vi "P4CMD Dialog - Project Options.vi"(6 "operation message":string, 8 "error in (no error)":errorcluster, 9 "configuration data in":string) -> (0 "error out":errorcluster, 1 "configuration data out":string, 5 "cancelled?":bool)   [LabVIEW 2017, in "NI_SCC_P4CMD.lvlib"]
uses:
  <vilib>/SourceControl/Providers/P4CMD/NI_SCC_P4CMD.lvlib
  <vilib>/SourceControl/support/SCCSup Dialog_GenMCLB_OnlineHelp.ctl
  <vilib>/SourceControl/Providers/P4CMD/P4CMD Operations.ctl
  <vilib>/SourceControl/support/SCCSup Dialog_GenMCLB_FilterParams.ctl
  <vilib>/SourceControl/support/SCCSup Message Strings GLBL.vi
panel:
  in  "P4Proj UIDialog FP Refs":T1
  in  "use defaults":bool=TRUE
  in  "browse clients":bool
  in  "browse users":bool
  in  "Client Workspace":string
  in  "Password":string
  in  "User":string
  in  "Port":string
  in  "Server":string
  in  "OK":bool
  in  "Cancel":bool
  in  "Help":bool
  # "1"
  # "Connect to"
  # "2"
  # "Connect as"
  # "3"
  # "Open client workspace"
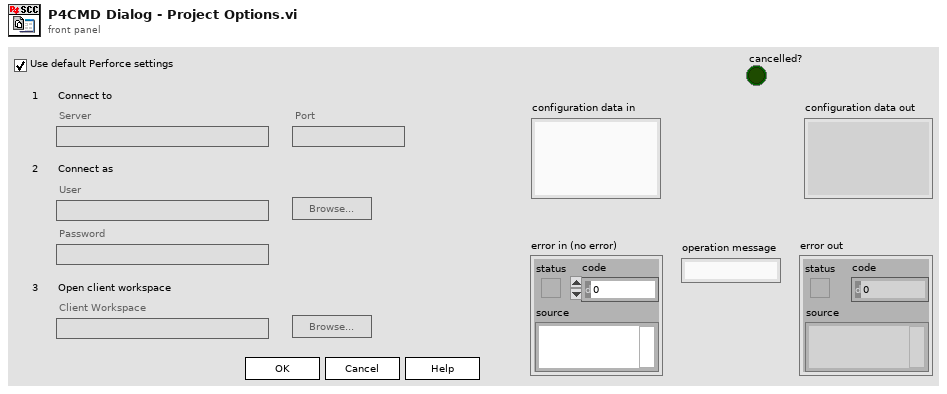
[diagram p1: front panel]
types:
  T1 = cluster{"browse users":refnum<vi>, "browse clients":refnum<vi>, "Server:":refnum<vi>, "Port:":refnum<vi>, "User:":refnum<vi>, "Password:":refnum<vi>, "Client Workspace:":refnum<vi>, "use default":refnum<vi>, "OK":refnum<vi>}
  T2 = typedef "SCCSup Dialog_GenMCLB_OnlineHelp.ctl" = cluster{"Operation":enum16{"Contents", "Key", "Close"}, "String to search for":string, "Path to the help file":path}
  T3 = typedef "NI_SCC_P4CMD.lvlib/P4CMD Operations.ctl" = enum16{"get all clients", "get all users", "describe changelist", "sync from depot", "open for edit", "submit to depot", "revert", "add to depot", "remove from depot", "print files revisions", "compare client file", "print depot file contents", "list opened files", "get file info", "lock files", "edit changelist spec", "info", "set variables"}
  T4 = typedef "SCCSup Dialog_GenMCLB_FilterParams.ctl" = cluster{"checkbox visible?":bool, "boolean text":string, "filter string":string, "filter column":i32}
  T5 = enum32{"Invalid", "Standard", "Closed", "Hidden", "Minimized", "Maximized"}
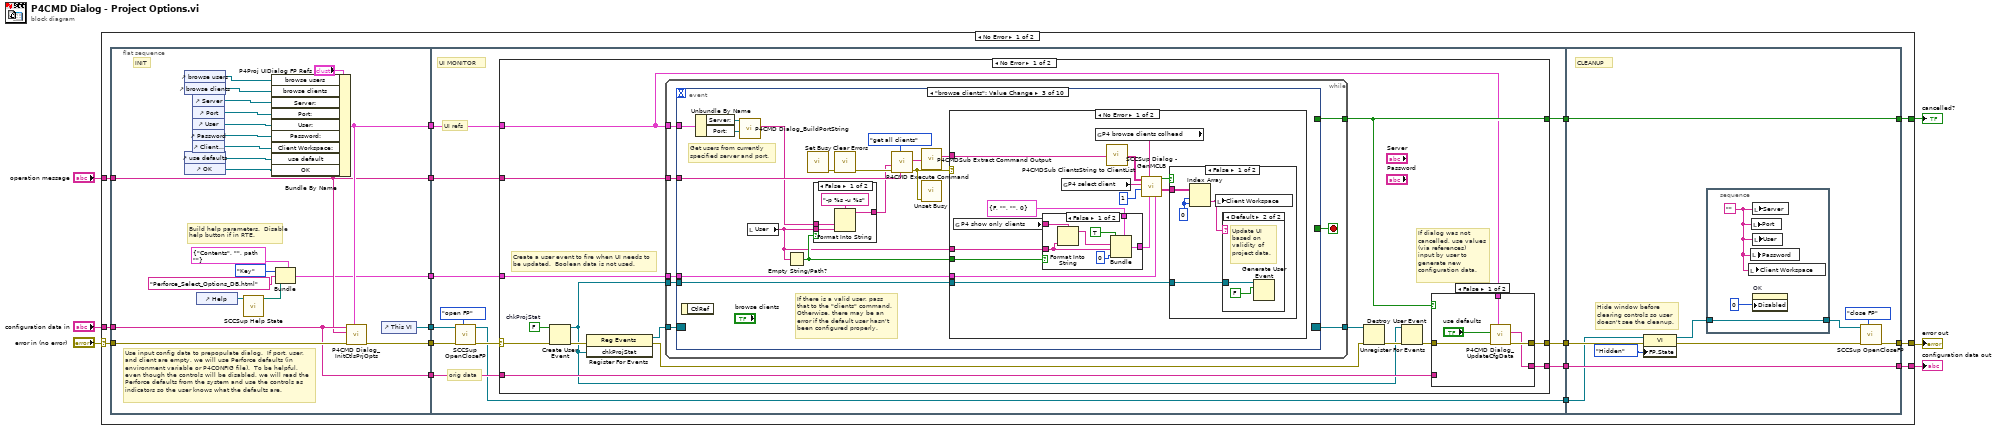
[diagram p0: block diagram]
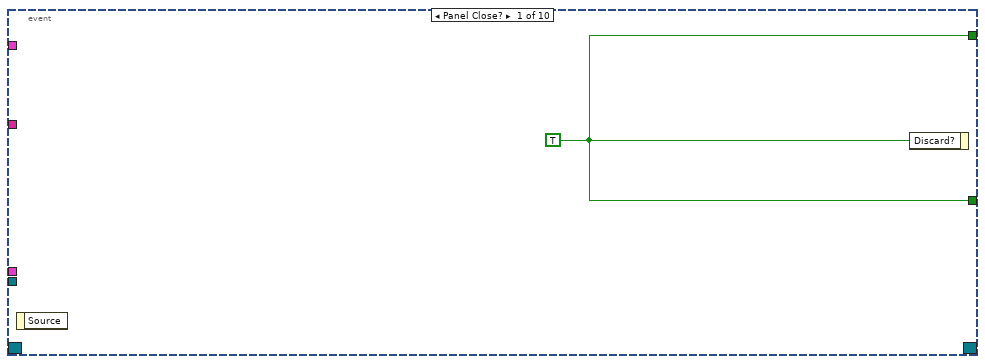
[diagram p3: hidden frame]
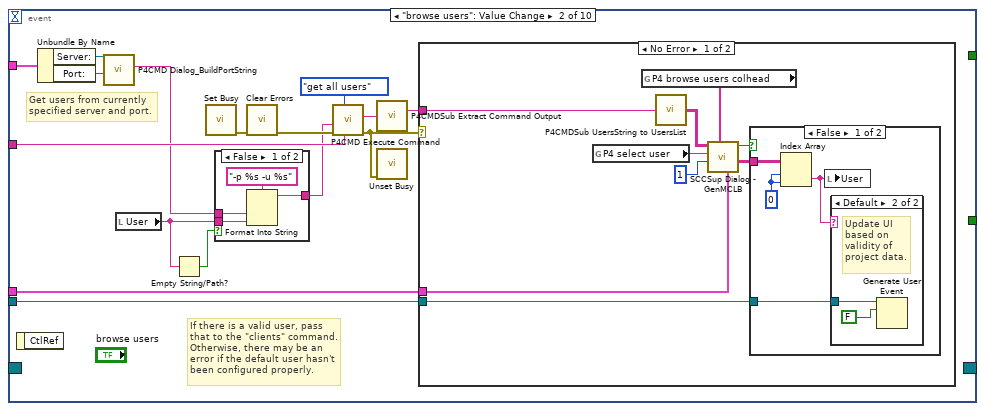
[diagram p4: hidden frame]
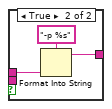
[diagram p5: hidden frame]
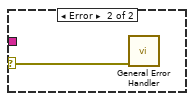
[diagram p8: hidden frame]
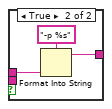
[diagram p9: hidden frame]
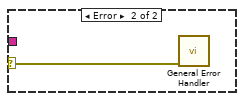
[diagram p13: hidden frame]
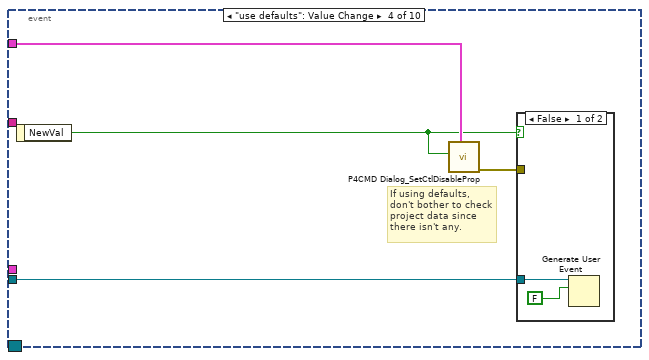
[diagram p14: hidden frame]
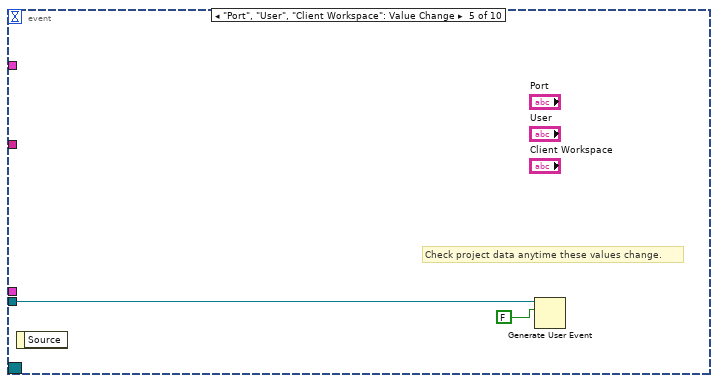
[diagram p16: hidden frame]
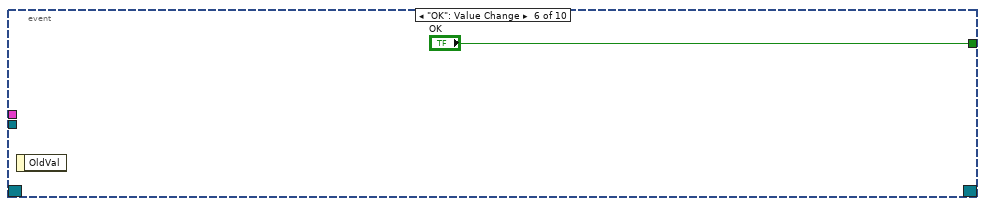
[diagram p17: hidden frame]
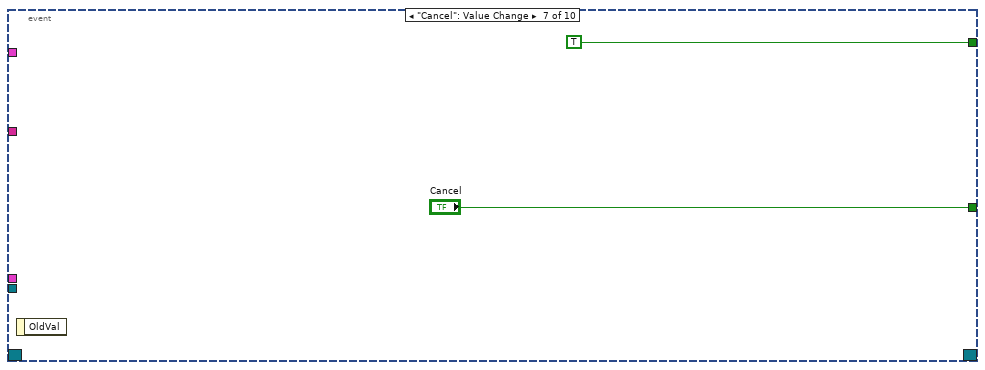
[diagram p18: hidden frame]
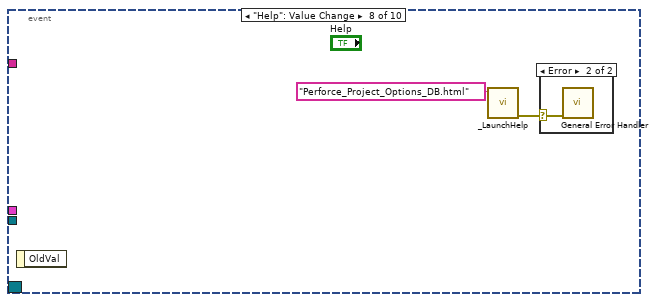
[diagram p19: hidden frame]
diagram:
  n1 = case shown="No Error" "error in (no error)" {
    selector: "error in (no error)" -> [w18 w219]
    tunnel: "configuration data in" -> [w19 w218]
    tunnel: [w16 w219] -> w4
    tunnel: [w14 w218] -> w3
    tunnel: "operation message" -> [w11 _]
    tunnel: [w9 _] -> w1
    frame No Error {
      n2 = flat-sequence {
        tunnel: [w29] -> w22
        tunnel: w18 -> [w36]
        tunnel: w19 -> [w33]
        tunnel: [w32] -> w21
        tunnel: [w33] -> w13
        tunnel: [w31] -> w12
        tunnel: w11 -> [w31]
        tunnel: [w30] -> w8
        tunnel: [w24] -> w7
        tunnel: [w48] -> w20
        tunnel: w22 -> [w55]
        tunnel: w21 -> [w54]
        tunnel: w8 -> [w53]
        tunnel: [w51] -> w17
        tunnel: [w49] -> w15
        tunnel: w13 -> [w50]
        tunnel: w12 -> [w47]
        tunnel: [w46] -> w10
        tunnel: w7 -> [w45]
        tunnel: w20 -> [w206]
        tunnel: w17 -> [w208]
        tunnel: [w213] -> w16
        tunnel: w15 -> [w212]
        tunnel: [w212] -> w14
        tunnel: [w211] -> w9
        tunnel: w10 -> [w211]
        frame #0 {
          # "Build help parameters.  Disable help button if in RTE."
          # "INIT"
          # "Use input config data to prepopulate dialog.  If port, user, and client are empty, we will use Perforce defaults (in environment variable or P4CONFIG file).  To be helpful, even though the controls will be disabled, we will read the Perforce defaults from the system and use the controls as indicators so the user knows what the defaults are."
          n3 = control-ref of="browse users"() -> (w43:refnum<vi>)
          n4 = control-ref of="browse clients"() -> (w42:refnum<vi>)
          n5 = control-ref of="use defaults"() -> (w35:refnum<vi>)
          n6 = control-ref of="OK"() -> (w34:refnum<vi>)
          n7 = control-ref of="Server"() -> (w41:refnum<vi>)
          n8 = control-ref of="Port"() -> (w40:refnum<vi>)
          n9 = control-ref of="User"() -> (w39:refnum<vi>)
          n10 = control-ref of="Password"() -> (w38:refnum<vi>)
          n11 = control-ref of="Client Workspace"() -> (w37:refnum<vi>)
          n12 = control-ref of="Help"() -> (w23:refnum<vi>)
          n13 = call <vilib>:"SCCSup Help State.vi"("help ref"=w23) -> ("lvdialog path"=w25:path)  [unwired: 10 in]
          n14 = Bundle By Name(cluster="P4Proj UIDialog FP Refs", "browse users"=w43, "browse clients"=w42, "Server:"=w41, "Port:"=w40, "User:"=w39, "Password:"=w38, "Client Workspace:"=w37, "use default"=w35, "OK"=w34) -> (w32:T1)
          n15 = Bundle(cluster=T2 {"Operation"=enum."Contents", "String to search for"="", "Path to the help file"=path ""} ("online help"), "Operation"=enum16{"Contents", "Key", "Close"}."Key", "String to search for"="Perforce_Select_Options_DB.html", "Path to the help file"=w25) -> (w24:T2)
          n16 = call <vilib>:"P4CMD Dialog_InitCtlsPrjOpts.vi"("P4Proj UIDialog FP Refs"=w32, "error in (no error)"=w36, "operation message"=w31, "configuration data"=w33) -> ("error out"=w30:errorcluster)  [unwired: 7 in]
          n17 = control-ref of="This VI"() -> (w29:refnum<vi>)
        }
        frame #1 {
          # "UI MONITOR"
          # "orig data"
          # "UI refs"
          n18 = call <vilib>:"SCCSup OpenCloseFP.vi"("function"=enum16{"open FP", "close FP"}."open FP", "error in (no error)"=w53, "VI Refnum in"=w55) -> ("error out"=w52:errorcluster, "VI Refnum out"=w48:refnum<vi>)  [unwired: 7 in]
          n19 = case shown="No Error" w52 {
            selector: w52 -> [w65 w204]
            tunnel: w54 -> [w68 _]
            tunnel: [w72 _] -> w46
            tunnel: [w69 w204] -> w51
            tunnel: w50 -> [w71 w203]
            tunnel: [w70 w203] -> w49
            tunnel: w47 -> [w67 _]
            tunnel: w45 -> [w57 _]
            frame No Error {
              w66 = FALSE  # chkProjStat
              # "Create a user event to fire when UI needs to be updated.  Boolean data is not used."
              # "If dialog was not cancelled, use values (via references)  input by user to generate new configuration data."
              n20 = Create User Event(user event datatype=w66, error in=w65) -> (user event=w58:refnum<user-event>, error out=w64:errorcluster)
              n21 = register-events(error in=w64, w58) -> (reference out=w63:refnum<event-registration>, error out=w61:errorcluster)  [unwired: 1 in]
              n22 = while {
                tunnel: [w86] -> w72
                tunnel: w68 -> [w85]
                tunnel: w67 -> [w84]
                tunnel: w63 -> [w83]
                tunnel: w58 -> [w82]
                tunnel: [w81] -> w62
                tunnel: w57 -> [w80]
                stop <- w87 stop-if-true
                n23 = event shown="[2] \"browse clients\": Value Change" {
                  selector: w83 -> [_ _ _ _ _ _ _ _ _ _]
                  dyn-events: [_ _ _ _ _ _ _ _ _ _] -> w81
                  timeout: _ -> [_ _ _ _ _ _ _ _ _ _]
                  tunnel: [w88 _ _ _ _ "OK" "Cancel" _ _ _] -> w87
                  tunnel: [w88 _ _ _ _ _ TRUE _ _ _] -> w86
                  tunnel: w85 -> [_ w101 w140 w183 _ _ _ _ _ w202]
                  tunnel: w84 -> [_ w100 w139 _ _ _ _ _ _ _]
                  tunnel: w82 -> [_ w96 w135 w180 w187 _ _ _ _ _]
                  tunnel: w80 -> [_ w93 w128 _ _ _ _ _ _ _]
                  event Panel Close? {
                    w88 = TRUE
                    n24 = event-data() -> ()  [unwired: 1 in, 1 out]
                    n25 = event-data("Discard?"=w88) -> ()  [unwired: 1 in, 1 out]
                  }
                  event "browse users": Value Change {
                    # "If there is a valid user, pass that to the \"clients\" command.  Otherwise, there may be an error if the default user hasn't been configured properly."
                    # "Get users from currently specified server and port."
                    n26 = event-data() -> ()  [unwired: 1 in, 1 out]
                    n27 = Unbundle By Name(w101) -> ("Server:"=w103:refnum<vi>, "Port:"=w102:refnum<vi>)
                    n28 = call <vilib>:"P4CMD Dialog_BuildPortString.vi"("Port:"=w102, "Server:"=w103) -> ("port string"=w92:string)  [unwired: 9 in]
                    n29 = local read "User"() -> (w91:string)
                    n30 = Empty String/Path?(string/path=w91) -> (empty?=w90:bool)
                    n31 = call <vilib>:"Set Busy.vi"() -> ("error out"=w99:errorcluster)  [unwired: 10 in, 1 out]
                    n32 = case shown="False" w90 {
                      tunnel: [w107 w110] -> w89
                      tunnel: w92 -> [w106 w109]
                      tunnel: w91 -> [w105 _]
                      frame False {
                        n33 = Format Into String(format string="-p %s -u %s", w106, w105) -> (resulting string=w107:string)  [unwired: 2 in, 1 out]
                      }
                      frame True {
                        n34 = Format Into String(format string="-p %s", w109) -> (resulting string=w110:string)  [unwired: 2 in, 1 out]
                      }
                    }
                    n35 = call <vilib>:"Clear Errors.vi"("error in (no error)"=w99) -> ("error out"=w97:errorcluster)  [unwired: 5 in, 1 out]
                    n36 = call <vilib>:"P4CMD Execute Command.vi"("operation message"=w100, "p4 operation"=P4CMD_Operations."get all users", "error in (no error)"=w97, "input string"=w89) -> ("error out"=w98:errorcluster, "command information"=w95:string)  [unwired: 5 in, 1 out]
                    n37 = call <vilib>:"P4CMDSub Extract Command Output.vi"("bundled message"=w95) -> ("command output"=w94:string)  [unwired: 13 in, 1 out]
                    n38 = call <vilib>:"Unset Busy.vi"("error in (no error)"=w98) -> ()  [unwired: 10 in, 1 out]
                    n39 = case shown="No Error" w98 {
                      selector: w98 -> [_ w127]
                      tunnel: w94 -> [w117 _]
                      tunnel: w96 -> [w115 _]
                      tunnel: w93 -> [w112 _]
                      frame No Error {
                        n40 = global read "SCCSup Message Strings GLBL.vi" "P4 select user"() -> (w113:string)
                        n41 = global read "SCCSup Message Strings GLBL.vi" "P4 browse users colhead"() -> (w114:string[])
                        n42 = call <vilib>:"P4CMDSub UsersString to UsersList.vi"("users string"=w117) -> ("users list"=w120:string[][])
                        n43 = call <vilib>:"SCCSup Dialog - GenMCLB.vi"("online help"=w112, "column header strings"=w114, "listbox selection mode"=1, "dialog title"=w113, "complete item names"=w120) -> ("selection"=w116:string[][], "cancelled?"=w118:bool)  [unwired: 5 in]
                        n44 = case shown="False" w118 {
                          tunnel: w116 -> [w124 _]
                          tunnel: w115 -> [w121 _]
                          frame False {
                            w123 = 0 ("index (row)")
                            n45 = Index Array(array=w124, index (row)=w123, index (col)=w123) -> (element=w122:string)
                            n46 = local write "User"(w122) -> ()
                            n47 = case shown="Default" w122 {
                              tunnel: w121 -> [_ w126]
                              frame "" {
                                # "Don't update if value is empty.  This is just in case."
                              }
                              frame Default {
                                # "Update UI based on validity of project data."
                                n48 = Generate User Event(user event=w126, event data cluster=FALSE ("event data")) -> ()  [unwired: 2 in, 2 out]
                              }
                            }
                          }
                          frame True {
                          }
                        }
                      }
                      frame Error {
                        n49 = call <vilib>:"General Error Handler.vi"("error in (no error)"=w127) -> ()  [unwired: 10 in, 5 out]
                      }
                    }
                  }
                  event "browse clients": Value Change {
                    # "If there is a valid user, pass that to the \"clients\" command.  Otherwise, there may be an error if the default user hasn't been configured properly."
                    # "Get users from currently specified server and port."
                    n50 = event-data() -> ()  [unwired: 1 in, 1 out]
                    n51 = Unbundle By Name(w140) -> ("Server:"=w142:refnum<vi>, "Port:"=w141:refnum<vi>)
                    n52 = call <vilib>:"P4CMD Dialog_BuildPortString.vi"("Port:"=w141, "Server:"=w142) -> ("port string"=w130:string)  [unwired: 9 in]
                    n53 = local read "User"() -> (w129:string)
                    n54 = Empty String/Path?(string/path=w129) -> (empty?=w132:bool)
                    n55 = call <vilib>:"Set Busy.vi"() -> ("error out"=w138:errorcluster)  [unwired: 10 in, 1 out]
                    n56 = case shown="False" w132 {
                      tunnel: [w146 w149] -> w131
                      tunnel: w130 -> [w145 w148]
                      tunnel: w129 -> [w144 _]
                      frame False {
                        n57 = Format Into String(format string="-p %s -u %s", w145, w144) -> (resulting string=w146:string)  [unwired: 2 in, 1 out]
                      }
                      frame True {
                        n58 = Format Into String(format string="-p %s", w148) -> (resulting string=w149:string)  [unwired: 2 in, 1 out]
                      }
                    }
                    n59 = call <vilib>:"Clear Errors.vi"("error in (no error)"=w138) -> ("error out"=w137:errorcluster)  [unwired: 5 in, 1 out]
                    n60 = call <vilib>:"P4CMD Execute Command.vi"("operation message"=w139, "p4 operation"=P4CMD_Operations."get all clients", "error in (no error)"=w137, "input string"=w131) -> ("error out"=w136:errorcluster, "command information"=w134:string)  [unwired: 5 in, 1 out]
                    n61 = call <vilib>:"P4CMDSub Extract Command Output.vi"("bundled message"=w134) -> ("command output"=w133:string)  [unwired: 13 in, 1 out]
                    n62 = call <vilib>:"Unset Busy.vi"("error in (no error)"=w136) -> ()  [unwired: 10 in, 1 out]
                    n63 = case shown="No Error" w136 {
                      selector: w136 -> [_ w179]
                      tunnel: w133 -> [w161 _]
                      tunnel: w135 -> [w157 _]
                      tunnel: w132 -> [w153 _]
                      tunnel: w129 -> [w152 _]
                      tunnel: w128 -> [w151 _]
                      frame No Error {
                        n64 = global read "SCCSup Message Strings GLBL.vi" "P4 show only clients"() -> (w154:string)
                        n65 = case shown="False" w153 {
                          tunnel: w152 -> [w168 _]
                          tunnel: [w171 w172] -> w159
                          tunnel: w154 -> [w167 _]
                          tunnel: T4 {"checkbox visible?"=FALSE, "boolean text"="", "filter string"="", "filter column"=0} ("filter parameters") -> [w165 w172]
                          frame False {
                            n66 = Format Into String(format string=w167, w168) -> (resulting string=w166:string)  [unwired: 2 in, 1 out]
                            n67 = Bundle(cluster=w165, "checkbox visible?"=TRUE, "boolean text"=w166, "filter string"=w168, "filter column"=0) -> (w171:T4)
                          }
                          frame True {
                          }
                        }
                        n68 = global read "SCCSup Message Strings GLBL.vi" "P4 select client"() -> (w156:string)
                        n69 = global read "SCCSup Message Strings GLBL.vi" "P4 browse clients colhead"() -> (w155:string[])
                        n70 = call <vilib>:"P4CMDSub ClientsString to ClientList.vi"("users string"=w161) -> ("users list"=w164:string[][])
                        n71 = call <vilib>:"SCCSup Dialog - GenMCLB.vi"("online help"=w151, "filter parameters"=w159, "column header strings"=w155, "listbox selection mode"=1, "dialog title"=w156, "complete item names"=w164) -> ("selection"=w160:string[][], "cancelled?"=w162:bool)  [unwired: 4 in]
                        n72 = case shown="False" w162 {
                          tunnel: w160 -> [w175 _]
                          tunnel: w157 -> [w173 _]
                          frame False {
                            w176 = 0 ("index (row)")
                            n73 = Index Array(array=w175, index (row)=w176, index (col)=w176) -> (element=w174:string)
                            n74 = local write "Client Workspace"(w174) -> ()
                            n75 = case shown="Default" w174 {
                              tunnel: w173 -> [_ w178]
                              frame "" {
                                # "Don't update if value is empty.  This is just in case."
                              }
                              frame Default {
                                # "Update UI based on validity of project data."
                                n76 = Generate User Event(user event=w178, event data cluster=FALSE ("event data")) -> ()  [unwired: 2 in, 2 out]
                              }
                            }
                          }
                          frame True {
                          }
                        }
                      }
                      frame Error {
                        n77 = call <vilib>:"General Error Handler.vi"("error in (no error)"=w179) -> ()  [unwired: 10 in, 5 out]
                      }
                    }
                  }
                  event "use defaults": Value Change {
                    # "If using defaults, don't bother to check project data since there isn't any."
                    n78 = event-data() -> ("NewVal"=w181:bool)  [unwired: 1 in]
                    n79 = call <vilib>:"P4CMD Dialog_SetCtlDisableProp.vi"("P4Proj UIDialog FP Refs"=w183, "use defaults?"=w181) -> ("error out"=w182:errorcluster)  [unwired: 9 in]
                    n80 = case shown="False" w181 {
                      tunnel: w182 -> [_ _]
                      tunnel: w180 -> [w185 _]
                      frame False {
                        n81 = Generate User Event(user event=w185, event data cluster=FALSE ("event data")) -> ()  [unwired: 2 in, 2 out]
                      }
                      frame True {
                      }
                    }
                  }
                  event "Port", "User", "Client Workspace": Value Change {
                    # "Check project data anytime these values change."
                    n82 = event-data() -> ()  [unwired: 1 in, 1 out]
                    n83 = Generate User Event(user event=w187, event data cluster=FALSE ("event data")) -> ()  [unwired: 2 in, 2 out]
                  }
                  event "OK": Value Change {
                    n84 = event-data() -> ()  [unwired: 1 in, 1 out]
                  }
                  event "Cancel": Value Change {
                    n85 = event-data() -> ()  [unwired: 1 in, 1 out]
                  }
                  event "Help": Value Change {
                    n86 = event-data() -> ()  [unwired: 1 in, 1 out]
                    n87 = call <helpdir>:"_LaunchHelp.vi"("HTML filename"="Perforce_Project_Options_DB.html" ("Help topic")) -> ("error out"=w192:errorcluster)  [unwired: 6 in]
                    n88 = case shown="Error" w192 {
                      selector: w192 -> [_ w193]
                      frame No Error {
                      }
                      frame Error {
                        n89 = call <vilib>:"General Error Handler.vi"("error in (no error)"=w193) -> ()  [unwired: 10 in, 5 out]
                      }
                    }
                  }
                  event Key Down? {
                    # "discard undo and redo"
                    n90 = event-data() -> ("Char"=w196:i16, "Mods.Menu Key"=w195:bool)  [unwired: 1 in]
                    n91 = Equal?(x=i16 122, y=w196) -> (x = y?=w199:bool)
                    n92 = Equal?(x=i16 90, y=w196) -> (x = y?=w198:bool)
                    n93 = Or(x=w198, y=w199) -> (x .or. y?=w197:bool)
                    n94 = And(x=w197, y=w195) -> (x .and. y?=w194:bool)
                    n95 = event-data("Discard?"=w194) -> ()  [unwired: 1 in, 1 out]
                  }
                  event User Event {
                    # "If the project data is invalid or empty, disable OK button.  If port is empty, disable Browse buttons since we use this value to read the clients and users.   If \"User\" control is empty, don't enable browsing clients"
                    n96 = event-data() -> ()  [unwired: 1 in, 1 out]
                    n97 = call <vilib>:"P4CMD Dialog_CheckProjData.vi"("P4Proj UIDialog FP Refs"=w202) -> ()  [unwired: 10 in, 1 out]
                  }
                }
              }
              n98 = Unregister For Events(event registration refnum=w62, error in=w61) -> (error out=w60:errorcluster)
              n99 = Destroy User Event(user event=w58, error in=w60) -> (error out=w59:errorcluster)
              n100 = case shown="False" w72 {
                tunnel: w71 -> [_ w79]
                tunnel: [w74 w79] -> w70
                tunnel: w59 -> [w77 w78]
                tunnel: [w76 w78] -> w69
                tunnel: w68 -> [w75 _]
                frame False {
                  n101 = call <vilib>:"P4CMD Dialog_UpdateCfgData.vi"("P4Proj UIDialog FP Refs"=w75, "error in (no error)"=w77, "use defaults?"="use defaults") -> ("error out"=w76:errorcluster, "config data out"=w74:string)  [unwired: 7 in]
                }
                frame True {
                }
              }
            }
            frame Error {
            }
          }
        }
        frame #2 {
          # "Hide window before clearing controls so user doesn't see the cleanup."
          # "CLEANUP"
          n102 = property class="VI"(reference=w206, error in=w208, "FP.State"=T5."Hidden" ("Front Panel Window:State")) -> (reference out=w205:refnum<vi>, error out=w207:errorcluster)
          n103 = stacked-sequence {
            tunnel: w205 -> [w215]
            tunnel: [w215] -> w210
            frame #0 {
              w217 = ""
              n104 = local write "Client Workspace"(w217) -> ()
              n105 = local write "Password"(w217) -> ()
              n106 = local write "Port"(w217) -> ()
              n107 = local write "Server"(w217) -> ()
              n108 = local write "User"(w217) -> ()
              n109 = property on="OK" class="Bool"("Disabled"=u8 0) -> ()  [unwired: 2 in, 2 out]
            }
          }
          n110 = call <vilib>:"SCCSup OpenCloseFP.vi"("function"=enum16{"open FP", "close FP"}."close FP", "error in (no error)"=w207, "VI Refnum in"=w210) -> ("error out"=w213:errorcluster)  [unwired: 7 in, 1 out]
        }
      }
    }
    frame Error {
    }
  }
  "error out" <- w4
  "configuration data out" <- w3
  "cancelled?" <- w1
